vi "Focus Fiducial.vi"(8 "error in":errorcluster, 10 "Component In":T1, 11 "Gantry In":refnum<k24>) -> (0 "error out":errorcluster, 2 "Component Out":T1, 3 "Gantry Out":refnum<k24>)   [LabVIEW 2021, in "Component Tray.lvclass"]
uses:
  Component/Component Tray.lvclass
  C:/Program Files (x86)/Aerotech/A3200/LabVIEW/2010/Bin/Aerotech.A3200.dll
  Program Files (x86)/Aerotech/A3200/LabVIEW/2010/Bin/Aerotech.A3200.dll
  Component/Find Component.ctl
  Controller/Camera/Machine Vision.ctl
  Controller/Camera/Camera.lvclass
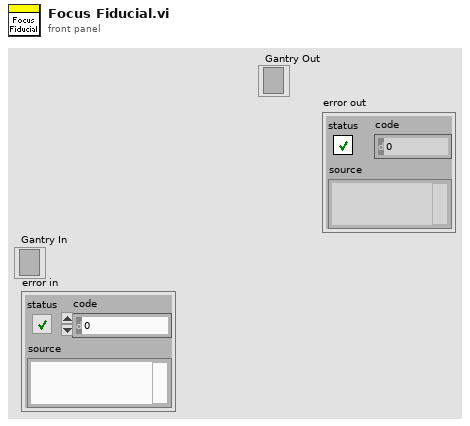
[diagram p1: front panel]
types:
  T1 = typedef "Component Tray.lvclass/Find Component.ctl" = cluster{"New Fiducials":dbl[], "Past Fiducials":dbl[][], "XYZTheta":dbl[], "Fiducials Path":path, "Position":i32, "CH1 Location":dbl[], "Sensor ID Location":dbl[], "initial rotation":dbl[], "CH2 location":dbl[], "max std variation":dbl, "max strength":dbl, "CH2 pattern matching":T2, "Fiducial Circle":T2, "Get Edge":T2, "Pos multiplier":dbl, "time to wait":u32, "fiducial to edge":dbl, "Protomodule?":bool, "Assembly Type":string, "CH1 to CH2":dbl, "Tray Number":string, "fiducial radius":dbl, "4 fiducials?":bool, "CH1 check":T2, "Edge Scan":T2, "CH1 pattern matching":T2, "Sensor Thickness":dbl}
  T2 = typedef "Camera.lvclass/Machine Vision.ctl" = enum16{"None", "Assembly Tray Circle", "Assembly Tray Fiducial", "Partial Hexaboard", "sensor edge init", "HB edge init", "sensor edge pos1", "sensor edge pos2", "HB edge pos1", "HB edge pos2", "Sensor CH1-2", "HB CH1", "HB CH2", "V3 Sensor Circle", "Hexaboard Circle", "sensor CH1 check", "HB CH1 check "}
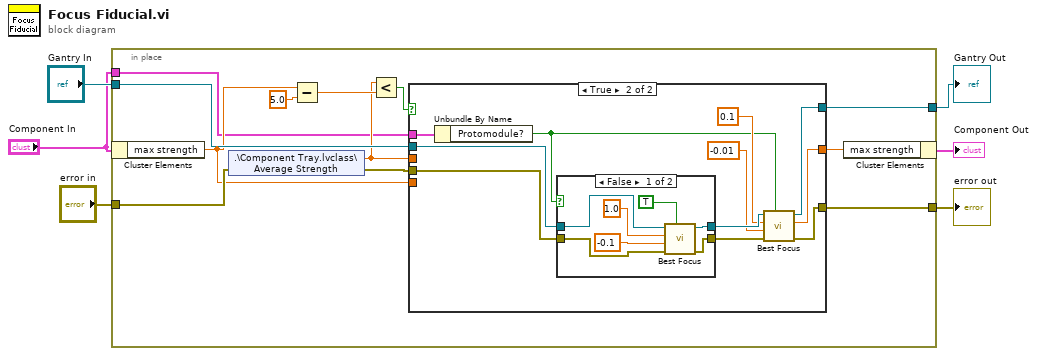
[diagram p0: block diagram]
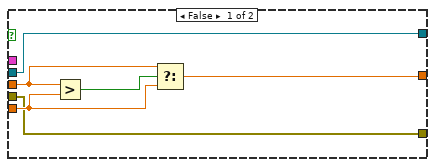
[diagram p2: hidden frame]
diagram:
  n1 = in-place {
    in-place-border: "Gantry In" -> [w18]
    in-place-border: "error in" -> [w13]
    in-place-border: [w17] -> w4
    in-place-border: [w16] -> w3
    in-place-border: "Component In" -> [w7]
    n2 = in-place-cluster #1("Component In") -> ("max strength"=w9:dbl)
    n3 = shared-variable ".\\Component Tray.lvclass\\Average Strength"(error in=w13) -> (w10:dbl, error out=w12:errorcluster)
    n4 = Subtract(x=w9, y=5.0) -> (x-y=w14:dbl)
    n5 = Less?(x=w10, y=w14) -> (x < y?=w11:bool)
    n6 = case shown="True" w11 {
      tunnel: w18 -> [w20 w35]
      tunnel: [w20 w33] -> w17
      tunnel: [w19 w32] -> w16
      tunnel: w12 -> [w19 w34]
      tunnel: w10 -> [w23 _]
      tunnel: w9 -> [w22 _]
      tunnel: [w21 w31] -> w8
      tunnel: w7 -> [_ w30]
      frame False {
        n7 = Greater?(x=w23, y=w22) -> (0:w24:bool)
        n8 = Select(t=w23, s=w24, f=w22) -> (s? t:f=w21:dbl)
      }
      frame True {
        n9 = Unbundle By Name(w30) -> ("Protomodule?"=w25:bool)
        n10 = case shown="False" w25 {
          tunnel: w35 -> [w42 w44]
          tunnel: w34 -> [w41 w43]
          tunnel: [w38 w44] -> w29
          tunnel: [w37 w43] -> w28
          frame False {
            n11 = call "Best Focus.vi"("Use Strength?"=TRUE, "error in (no error)"=w41, "Inc by"=-0.1, "Start"=1.0, "Gantry In"=w42) -> ("error out"=w37:errorcluster, "Gantry Out"=w38:refnum<k24>)  [unwired: 4 in, 1 out]
          }
          frame True {
          }
        }
        n12 = call "Best Focus.vi"("Use Strength?"=w25, "error in (no error)"=w28, "Inc by"=-0.01, "Start"=0.1, "Gantry In"=w29) -> ("error out"=w32:errorcluster, "max value"=w31:dbl, "Gantry Out"=w33:refnum<k24>)  [unwired: 4 in]
      }
    }
    n13 = in-place-cluster #1("max strength"=w8) -> (→"Component Out":T1)
  }
  "Gantry Out" <- w4
  "error out" <- w3
